vi "AutoRepScan.vi"() -> ()   [LabVIEW 2022 SP3]
uses:
  Control_AutoRepScan.ctl
  <vilib>/Utility/sysdir.llb/System Directory Type.ctl
  Peripherals/ActionEngineEnum(V2).ctl
  Peripherals/Control_ZurichAE.ctl
  <vilib>/DAQmx/read.llb/DAQmx Read (Counter U32 1Chan 1Samp).vi
  <vilib>/DAQmx/create/channels.llb/DAQmx Create Channel (CI-Count Edges).vi
  <vilib>/DAQmx/miscellaneous.llb/DAQmx Fill In Error Info.vi
  <resource>/objmgr/daqmx.rc
  C:/Users/mnopl/Desktop/Software/mnOPSuite/PRISM/Thorlabs.MotionControl.Controls.dll
  Thorlabs.MotionControl.Controls.dll
panel:
  in  "HeNe Vosc":cluster{"Node 1 (V)":dbl, "Node 2 (V)":dbl}={"Node 1 (V)"=0.04852, "Node 2 (V)"=0.07}
  in  "Do replicate on \"configure\"?":bool=TRUE
  out "Duration of scans":dbl(graph)=55.78836666666667
  in  "Timeout (min.)":dbl=1000.0
  out "PSHet V Oscillation vs. Wavelength":cluster{dbl[], dbl[]}(graph)={[3.16, 2.5200000000000005, 2.8400000000000003], [0.10222000000000002, 0.08074, 0.08074]}
  out "Current wavelength (microns)":dbl=2.8400000000000003
  in  "Replication wait time (s)":i32=2
  out "dWavelength/drep":dbl=0.32000000000000006
  in  "Default Zurich XY gain":dbl=100.0
  in  "Compromise Vosc to HeNeStab":bool=TRUE
  in  "Starting wavelength (microns)":dbl=2.2
  in  "Configure scan":bool
  out "Kinesis Errors":errorcluster
  out "dKinesis/dRep":dbl=0.010000000000000142
  in  "Ending Kinesis Pos.":dbl=12.38
  in  "Starting Kinesis Pos.":dbl=12.33
  in  "KCubeStepperControl":refnum<k24>(container)
  out "Scans Completed":bool
  in  "Manually increment counter":bool
  out "DAQ errors":errorcluster
  out "Digital counter":i32
  in  "Trigger Edge":i32(ring)=10171 items=["Rising"=10280, "Falling"=10171]
  in  "Scan (frame) trigger":tag="/Dev1/PFI1"
  in  "TTL control\nactive":bool
  out "Scans active":bool
  out "Python errors":errorcluster
  out "Zurich errors":errorcluster
  out "Current PSHet Osc":dbl=0.08074
  out "Number of scans":i32=3
  out "dOsc/drep":dbl=0.009600000000000001
  in  "Ending PSHet Osc":dbl=0.114
  in  "Starting PSHet Osc":dbl=0.066
  in  "Zurich Address":string="DEV1925"
  out "Latest alpha command":string="@rep load 2"
  out "# Scans completed":i32=3
  out "Current status":string="Awaiting command..."
  in  "Halt program":bool
  in  "Cancel Button":bool
  out "Time elapsed this scan (min)":dbl
  out "Time for last scan (min)":dbl
  in  "Current replication":i32=3
  in  "Execute Sequence":bool
  in  "Replicate to #":i32=5 min=0 max=49
  in  "Replicate from #":i32 min=0 max=49
  # "NOTE:  Replication list is assumed to increment uniformly in infrared *wavelength*, not uniformly in *frequency*."
  # "These should be a nearest pair of Vosc values at which HeNe-stab signal vanishes.\n(Updated 2025.05.08)"
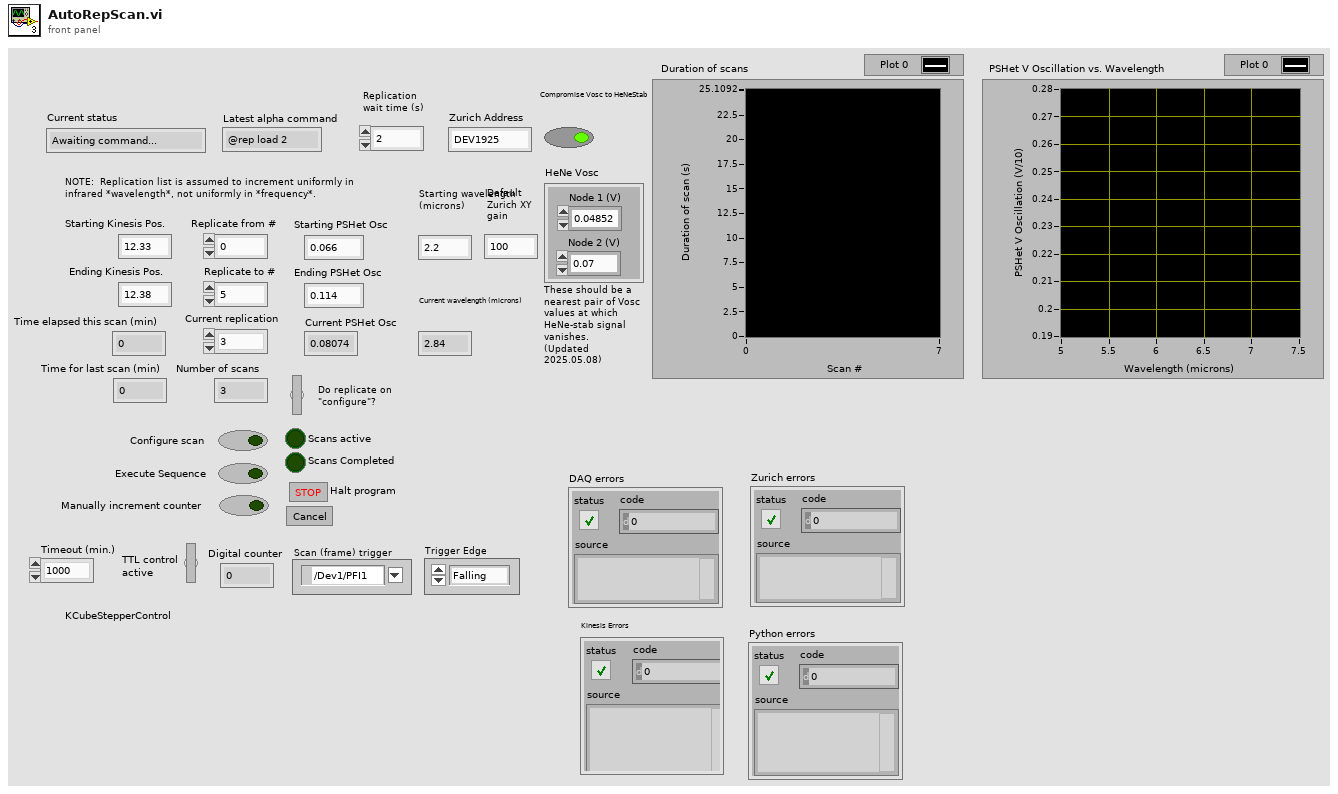
[diagram p1: front panel]
types:
  T1 = typedef "Control_ZurichAE.ctl" = enum16{"Initialize", "Set V oscillation", "Set XY gains", "Close", "Done"}
  T2 = typedef "ActionEngineEnum(V2).ctl" = enum16{"Open Connection", "IsSettingsInitialized? ", "Done", "Get Position", "Settings", "Home", "Move Absolute", "Move Relative", "Step", "Stop Action", "Close Connection"}
  T3 = typedef "System Directory Type.ctl" = i32
  T4 = typedef "Control_AutoRepScan.ctl" = enum16{"Sit Idle", "Configure scan", "Wait for scan", "Initialize", "Finalize", "Start DAQ control", "Poll DAQ control", "Stop DAQ control"}
  T5 = enum8{"Enabled", "Disabled", "Disabled and Grayed Out"}
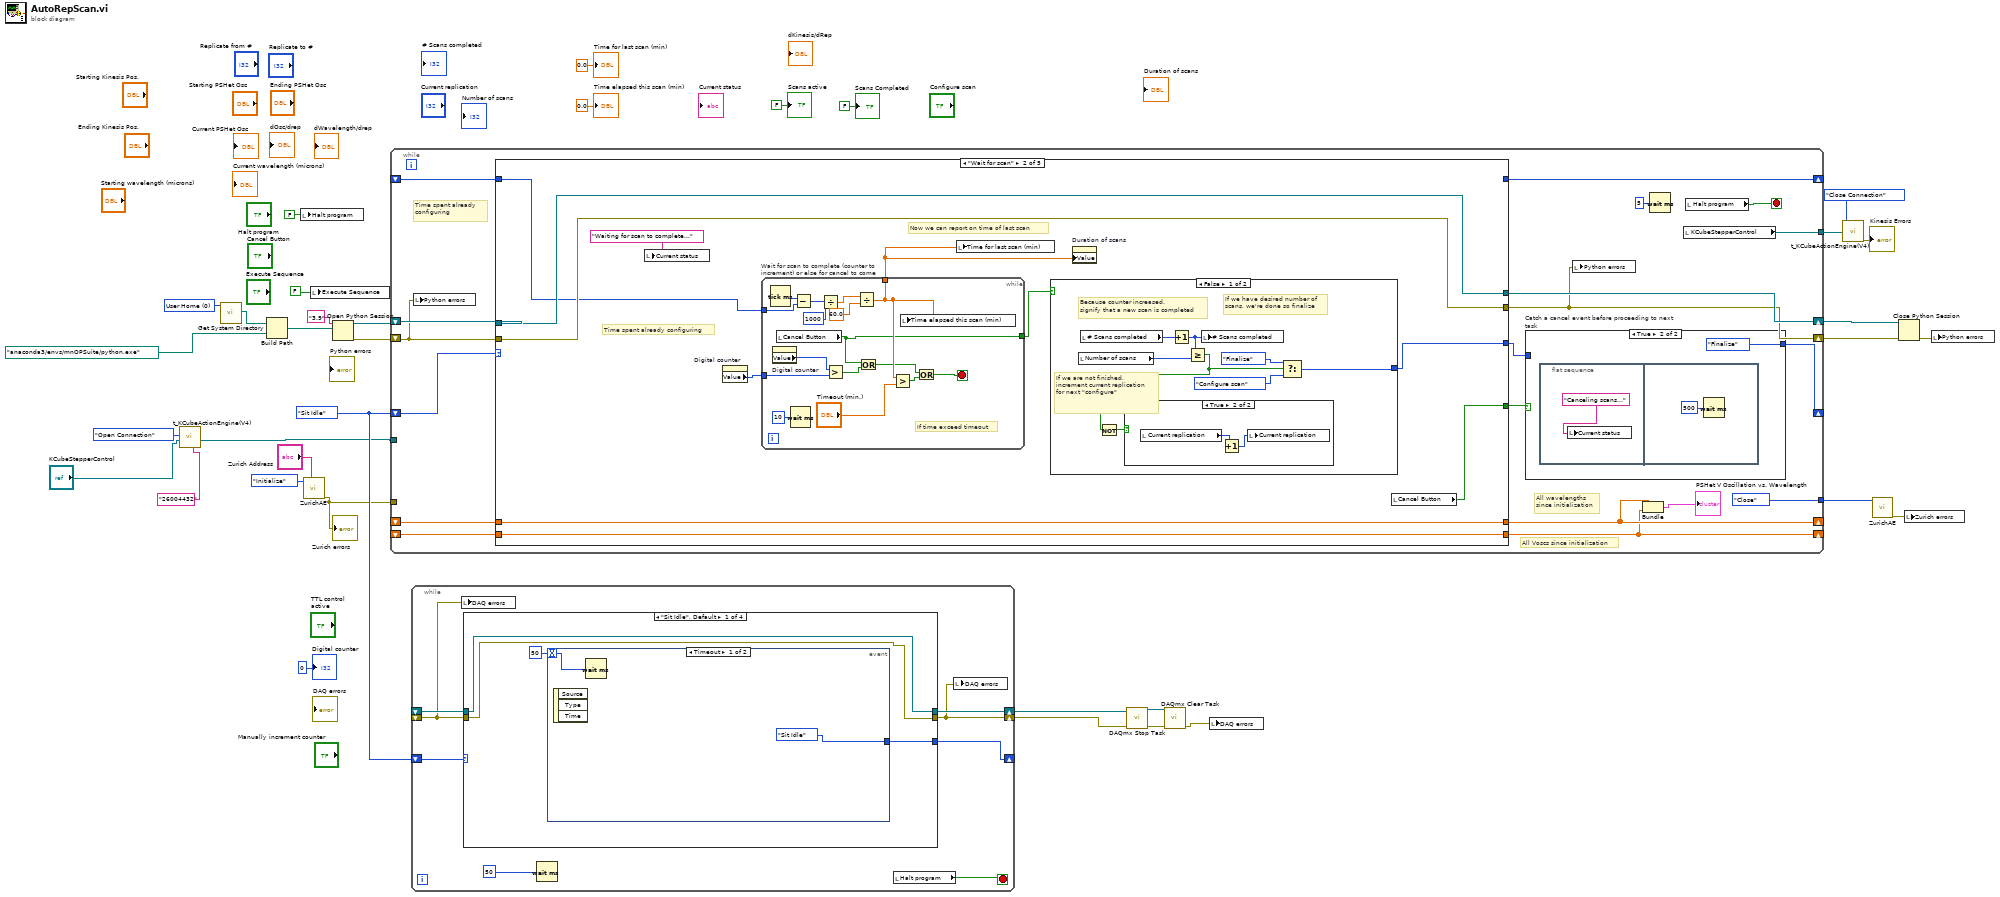
[diagram p0: block diagram]
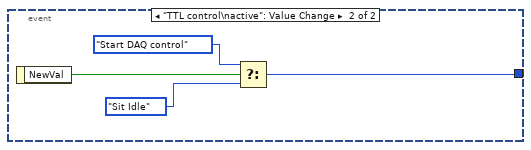
[diagram p2: hidden frame]
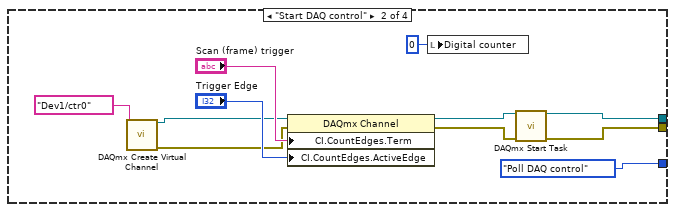
[diagram p3: hidden frame]
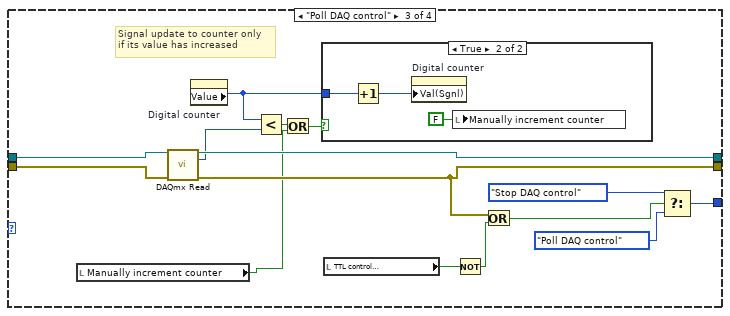
[diagram p4: hidden frame]
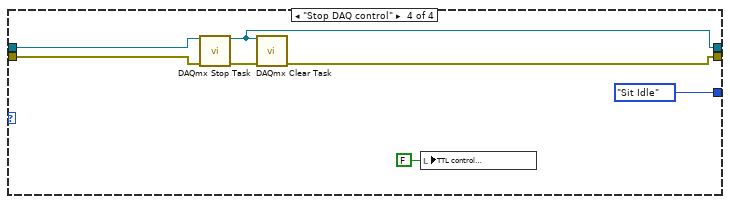
[diagram p6: hidden frame]
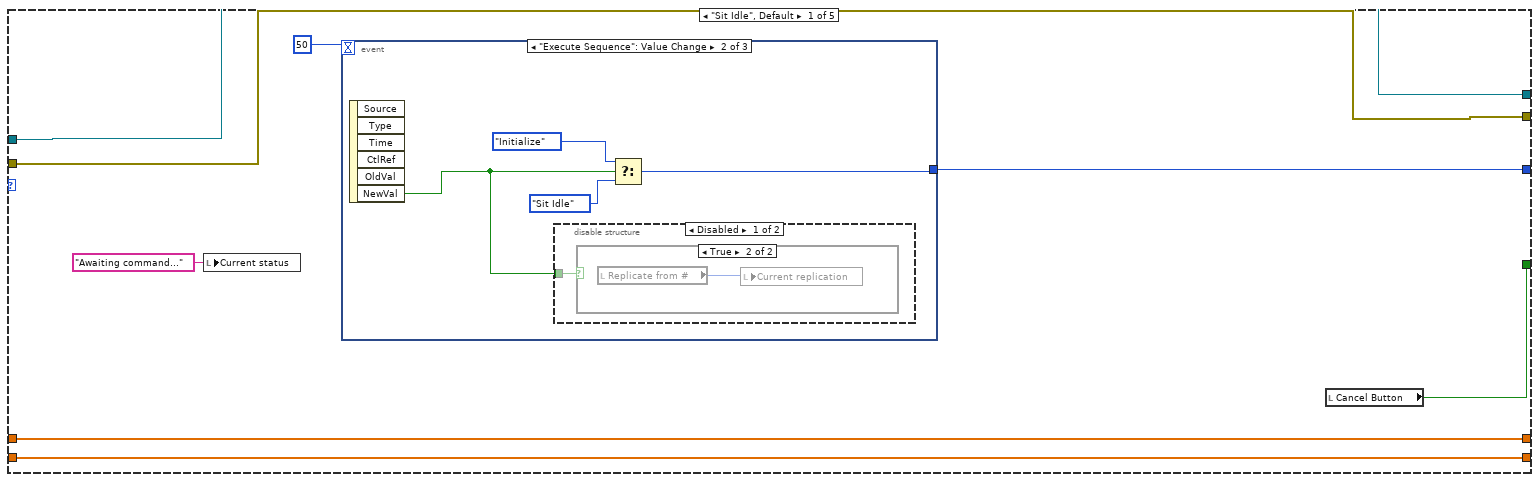
[diagram p8: hidden frame]
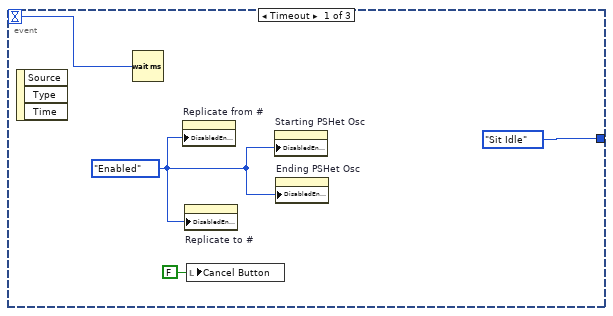
[diagram p9: hidden frame]
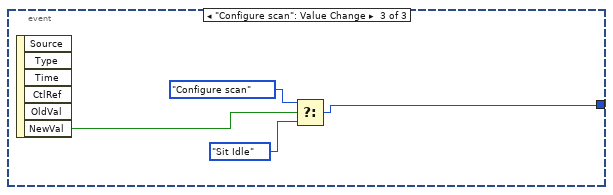
[diagram p12: hidden frame]
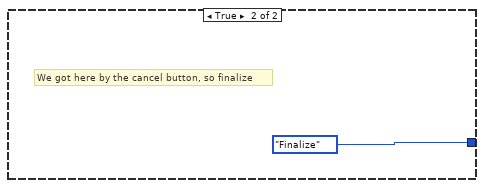
[diagram p14: hidden frame]
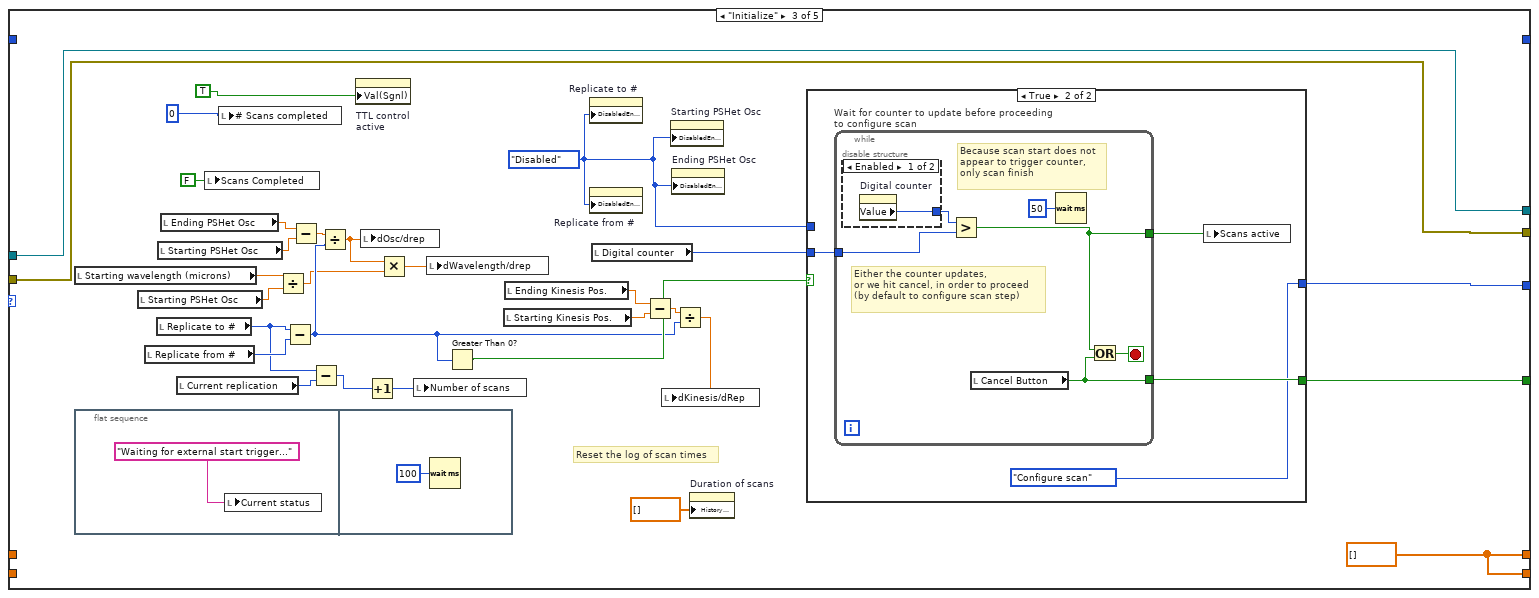
[diagram p15: hidden frame]
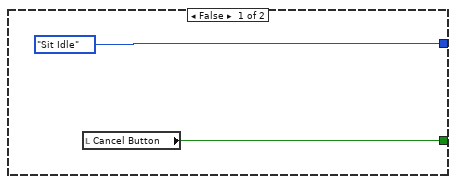
[diagram p16: hidden frame]
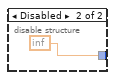
[diagram p17: hidden frame]
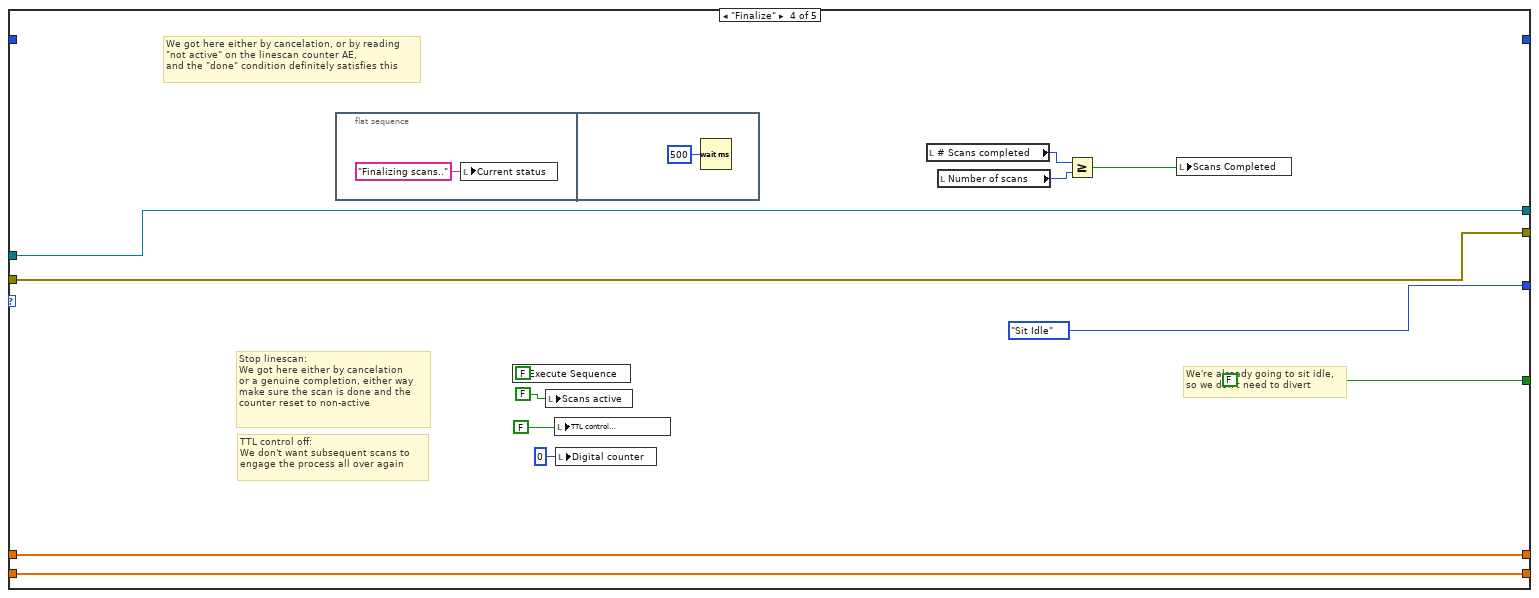
[diagram p18: hidden frame]
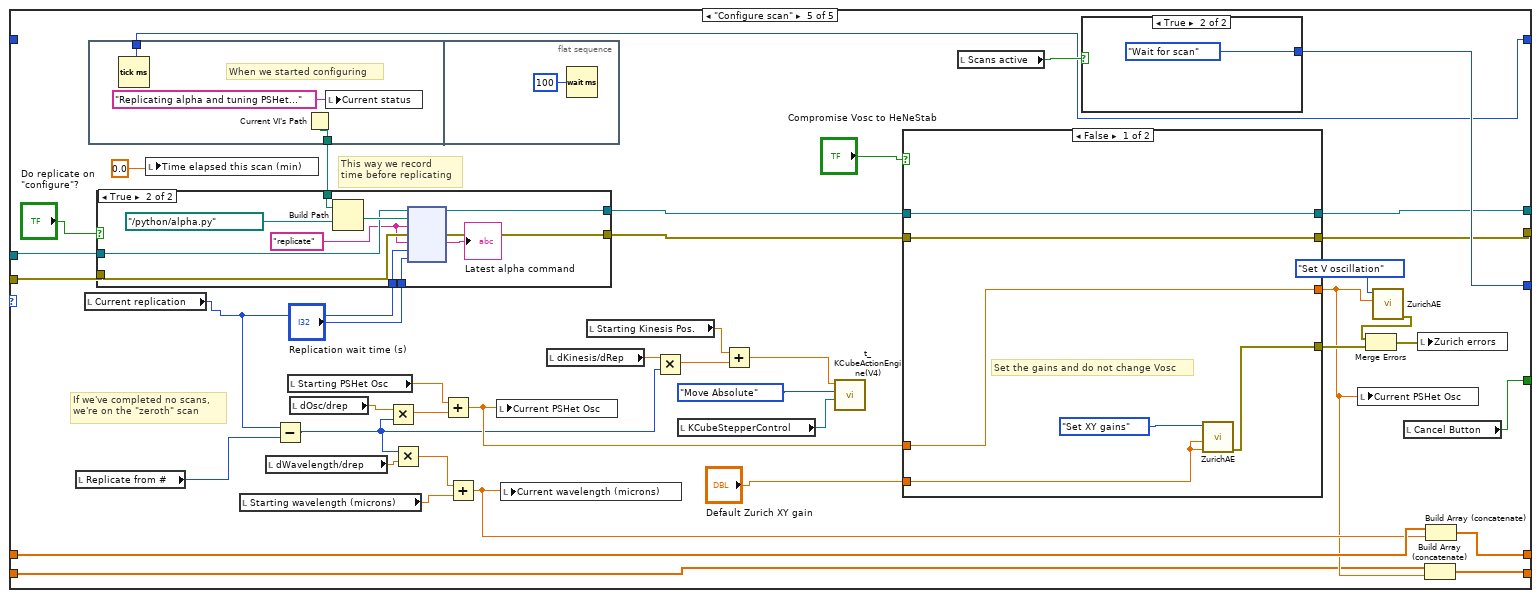
[diagram p19: hidden frame]
diagram:
  w34 = T3 0 items=["User Home"=0, "User Desktop"=1, "User Documents"=2, "User Application Data"=3, "User Preferences"=4, "User Temporary"=5, "Public Documents"=6, "Public Application Data"=7, "Public Preferences"=8, "Public Cache"=13, "System Core Libraries"=9, "System Installed Libraries"=10, "Application Files"=11, "Boot Volume Root"=12] ("system directory type")
  w23 = Control_AutoRepScan."Sit Idle"
  n1 = call "t_KCubeActionEngine(V4).vi"("SerialNumber"="26004432", "KCubeStepperControl"="KCubeStepperControl", "Action"=ActionEngineEnum(V2)."Open Connection") -> ("KCubeStepperControl Out"=w9:refnum<k24>)  [unwired: 5 in, 3 out]
  n2 = call <vilib>:"Get System Directory.vi"("system directory type"=w34) -> ("system directory"=w33:path)  [unwired: 10 in]
  n3 = Build Path(base path=w33, name or relative path=path "anaconda3/envs/mnOPSuite/python.exe") -> (appended path=w31:path)
  n4 = local write "Halt program"(FALSE ("Halt program")) -> ()
  n5 = call "ZurichAE.vi"("zi Address"="Zurich Address", "Action"=Control_ZurichAE."Initialize") -> ("Zurich Errors"=w3:errorcluster)  [unwired: 9 in]
  "Zurich errors" <- w3
  n6 = local write "Execute Sequence"(FALSE ("Execute")) -> ()
  n7 = Open Python Session(python version="3.9", python path=w31) -> (session out=w27:refnum<k35>, error out=w28:errorcluster)  [unwired: 1 in]
  n8 = while {
    shift-right: [w51] -> _
    shift-left: w23 -> [w54]
    shift-right: [w50] -> w30
    shift-left: w27 -> [w49]
    shift-right: [w46] -> w29
    shift-left: w28 -> [w47]
    tunnel: w9 -> [_]
    tunnel: [w44] -> w8
    tunnel: w3 -> [_]
    tunnel: [Control_ZurichAE."Close" ("Action")] -> w2
    shift-right: [w39] -> _
    shift-left: _ -> [w42]
    shift-right: [w38] -> _
    shift-left: _ -> [w41]
    shift-right: [w37] -> _
    shift-left: _ -> [w36]
    stop <- w53 stop-if-true
    # "Time spent already configuring"
    # "All Voscs since initialization"
    # "All wavelengths\nsince initialization"
    n9 = local write "Python errors"(w47) -> ()
    n10 = case shown="\"Wait for scan\"" w54 {
      tunnel: [w66 w85 w148 Control_AutoRepScan."Sit Idle" w216] -> w52
      tunnel: w47 -> [w63 w89 w140 w176 w220]
      tunnel: w49 -> [w64 w90 w141 w177 w221]
      tunnel: [w64 w90 w141 w177 w198] -> w50
      tunnel: [w63 w89 w140 w176 w196] -> w46
      tunnel: [w62 w91 w142 FALSE w215] -> w48
      tunnel: [w60 w84 w124 w166 w189] -> w39
      tunnel: [w59 w83 w124 w165 w186] -> w38
      tunnel: w42 -> [w60 w84 _ w166 w191]
      tunnel: w41 -> [w59 w83 _ w165 w187]
      tunnel: [_ _ _ _ w185] -> w37
      tunnel: w36 -> [_ w81 _ _ _]
      frame "Sit Idle", Default {
        n11 = local write "Current status"("Awaiting command..." ("Current status")) -> ()
        n12 = event shown="[1] \"Execute Sequence\": Value Change" {
          selector: _ -> [_ _ _]
          dyn-events: _ -> [_ _ _]
          timeout: 50 -> [w67 _ _]
          tunnel: [Control_AutoRepScan."Sit Idle" w73 w77] -> w66
          event Timeout {
            w69 = T5."Enabled" ("Disabled")
            n13 = event-data() -> ()  [unwired: 1 in, 3 out]
            n14 = Wait (ms)(milliseconds to wait=w67) -> ()  [unwired: 1 out]
            n15 = property on="Replicate from #" class="DigNum (strict)"("DisabledEnum"=w69) -> ()  [unwired: 2 in, 2 out]
            n16 = property on="Replicate to #" class="DigNum (strict)"("DisabledEnum"=w69) -> ()  [unwired: 2 in, 2 out]
            n17 = local write "Cancel Button"(FALSE ("Cancel Button")) -> ()
            n18 = property on="Starting PSHet Osc" class="DigNum (strict)"("DisabledEnum"=w69) -> ()  [unwired: 2 in, 2 out]
            n19 = property on="Ending PSHet Osc" class="DigNum (strict)"("DisabledEnum"=w69) -> ()  [unwired: 2 in, 2 out]
          }
          event "Execute Sequence": Value Change {
            n20 = event-data() -> ("NewVal"=w71:bool)  [unwired: 1 in, 5 out]
            n21 = disable-structure shown="Disabled" {
              disable-tunnel: w71 -> [w75 _]
              frame Disabled {
                n22 = case shown="True" w75 {
                  frame False {
                  }
                  frame True {
                    n23 = local read "Replicate from #"() -> (w76:i32)
                    n24 = local write "Current replication"(w76) -> ()
                  }
                }
              }
              frame Enabled {
              }
            }
            n25 = Select(t=Control_AutoRepScan."Initialize", s=w71, f=Control_AutoRepScan."Sit Idle") -> (s? t:f=w73:T4)
          }
          event "Configure scan": Value Change {
            n26 = event-data() -> ("NewVal"=w80:bool)  [unwired: 1 in, 5 out]
            n27 = Select(t=Control_AutoRepScan."Configure scan", s=w80, f=Control_AutoRepScan."Sit Idle") -> (s? t:f=w77:T4)
          }
        }
        n28 = local read "Cancel Button"() -> (w62:bool)
      }
      frame "Wait for scan" {
        # "Time spent already configuring"
        # "Now we can report on time of last scan"
        n29 = local write "Current status"("Waiting for scan to complete..." ("Current status")) -> ()
        n30 = property on="Digital counter" class="DigNum (strict)"() -> ("Value"=w87:i32)  [unwired: 2 in, 2 out]
        n31 = while "Wait for scan to complete (counter to increment) or else for cancel to come" {
          tunnel: w81 -> [w112]
          tunnel: [w108] -> w82
          tunnel: w87 -> [w115]
          tunnel: [w104] -> w86
          stop <- w106 stop-if-true
          # "If time exceed timeout"
          n32 = Tick Count (ms)() -> (millisecond timer value=w113:u32)
          n33 = property on="Digital counter" class="DigNum (strict)"() -> ("Value"=w116:i32)  [unwired: 2 in, 2 out]
          n34 = local read "Cancel Button"() -> (w104:bool)
          n35 = Wait (ms)(milliseconds to wait=u32 10) -> ()  [unwired: 1 out]
          n36 = Subtract(x=w113, y=w112) -> (x-y=w114:u32)
          n37 = Divide(x=w114, y=u32 1000) -> (x/y=w111:dbl)
          n38 = Greater?(x=w116, y=w115) -> (0:w105:bool)
          n39 = Divide(x=w111, y=60.0) -> (x/y=w108:dbl)
          n40 = Or(x=w104, y=w105) -> (x .or. y?=w107:bool)
          n41 = Greater?(x=w108, y="Timeout (min.)") -> (0:w109:bool)
          n42 = local write "Time elapsed this scan (min)"(w108) -> ()
          n43 = Or(x=w107, y=w109) -> (x .or. y?=w106:bool)
        }
        n44 = local write "Time for last scan (min)"(w82) -> ()
        n45 = case shown="False" w86 {
          tunnel: [w94 Control_AutoRepScan."Finalize"] -> w85
          frame False {
            # "If we are not finished, increment current replication for next \"configure\""
            # "If we have desired number of\nscans, we're done so finalize"
            # "Because counter increased,\nsignify that a new scan is completed"
            n46 = local read "Number of scans"() -> (w98:i32)
            n47 = local read "# Scans completed"() -> (w99:i32)
            n48 = Increment(x=w99) -> (x+1=w97:i32)
            n49 = Greater Or Equal?(x=w97, y=w98) -> (x >= y?=w93:bool)
            n50 = Not(x=w93) -> (.not. x?=w92:bool)
            n51 = case shown="True" w92 {
              frame False {
              }
              frame True {
                n52 = local read "Current replication"() -> (w100:i32)
                n53 = Increment(x=w100) -> (x+1=w101:i32)
                n54 = local write "Current replication"(w101) -> ()
              }
            }
            n55 = local write "# Scans completed"(w97) -> ()
            n56 = Select(t=Control_AutoRepScan."Finalize", s=w93, f=Control_AutoRepScan."Configure scan") -> (s? t:f=w94:T4)
          }
          frame True {
            # "We got here by the cancel button, so finalize"
          }
        }
        n57 = property on="Duration of scans" class="WFChart (strict)"("Value"=w82) -> ()  [unwired: 2 in, 2 out]
        n58 = local read "Cancel Button"() -> (w91:bool)
      }
      frame "Initialize" {
        w124 = dbl[] []
        w144 = T5."Disabled" ("Disabled")
        # "Reset the log of scan times"
        n59 = local read "Starting wavelength (microns)"() -> (w123:dbl)
        n60 = flat-sequence {
          frame #0 {
            n61 = local write "Current status"("Waiting for external start trigger..." ("Current status")) -> ()
          }
          frame #1 {
            n62 = Wait (ms)(milliseconds to wait=u32 100) -> ()  [unwired: 1 out]
          }
        }
        n63 = local read "Starting PSHet Osc"() -> (w129:dbl)
        n64 = local read "Replicate from #"() -> (w126:i32)
        n65 = local read "Replicate to #"() -> (w121:i32)
        n66 = local read "Starting PSHet Osc"() -> (w145:dbl)
        n67 = local read "Ending PSHet Osc"() -> (w146:dbl)
        n68 = local read "Current replication"() -> (w120:i32)
        n69 = local write "Scans Completed"(FALSE ("Scans Completed")) -> ()
        n70 = local write "# Scans completed"(0 ("# Scans completed")) -> ()
        n71 = Divide(x=w123, y=w129) -> (x/y=w128:dbl)
        n72 = Subtract(x=w121, y=w126) -> (x-y=w134:i32)
        n73 = Subtract(x=w146, y=w145) -> (x-y=w143:dbl)
        n74 = Subtract(x=w121, y=w120) -> (x-y=w119:i32)
        n75 = Divide(x=w143, y=w134) -> (x/y=w127:dbl)
        n76 = property on="TTL control\nactive" class="Bool (strict)"("Val(Sgnl)"=TRUE ("TTL control\nactive")) -> ()  [unwired: 2 in, 2 out]
        n77 = local write "dOsc/drep"(w127) -> ()
        n78 = Increment(x=w119) -> (x+1=w139:i32)
        n79 = Multiply(x=w127, y=w128) -> (x*y=w125:dbl)
        n80 = local write "Number of scans"(w139) -> ()
        n81 = local write "dWavelength/drep"(w125) -> ()
        n82 = Greater Than 0?(x=w134) -> (x > 0?=w147:bool)
        n83 = local read "Starting Kinesis Pos."() -> (w130:dbl)
        n84 = local read "Ending Kinesis Pos."() -> (w131:dbl)
        n85 = property on="Replicate to #" class="DigNum (strict)"("DisabledEnum"=w144) -> ()  [unwired: 2 in, 2 out]
        n86 = property on="Replicate from #" class="DigNum (strict)"("DisabledEnum"=w144) -> ()  [unwired: 2 in, 2 out]
        n87 = local read "Digital counter"() -> (w138:i32)
        n88 = Subtract(x=w131, y=w130) -> (x-y=w133:dbl)
        n89 = property on="Starting PSHet Osc" class="DigNum (strict)"("DisabledEnum"=w144) -> ()  [unwired: 2 in, 2 out]
        n90 = property on="Ending PSHet Osc" class="DigNum (strict)"("DisabledEnum"=w144) -> ()  [unwired: 2 in, 2 out]
        n91 = Divide(x=w133, y=w134) -> (x/y=w132:dbl)
        n92 = local write "dKinesis/dRep"(w132) -> ()
        n93 = property on="Duration of scans" class="WFChart (strict)"("History Data"=dbl[] []) -> ()  [unwired: 2 in, 2 out]
        n94 = case shown="True" w147 {
          tunnel: [Control_AutoRepScan."Sit Idle" Control_AutoRepScan."Configure scan"] -> w148
          tunnel: w144 -> [_ _]
          tunnel: [w151 w155] -> w142
          tunnel: w138 -> [_ w156]
          frame False {
            n95 = local read "Cancel Button"() -> (w151:bool)
          }
          frame True {
            n96 = while "Wait for counter to update before proceeding to configure scan" {
              tunnel: w156 -> [w161]
              tunnel: [w159] -> w155
              tunnel: [w157] -> w153
              stop <- w158 stop-if-true
              # "Because scan start does not\nappear to trigger counter, \nonly scan finish"
              # "Either the counter updates,\nor we hit cancel, in order to proceed\n(by default to configure scan step)"
              n97 = disable-structure shown="Enabled" {
                disable-tunnel: [w163 inf] -> w162
                frame Enabled {
                  n98 = property on="Digital counter" class="DigNum (strict)"() -> ("Value"=w163:i32)  [unwired: 2 in, 2 out]
                }
                frame Disabled {
                }
              }
              n99 = Greater?(x=w162, y=w161) -> (0:w157:bool)
              n100 = local read "Cancel Button"() -> (w159:bool)
              n101 = Wait (ms)(milliseconds to wait=u32 50) -> ()  [unwired: 1 out]
              n102 = Or(x=w157, y=w159) -> (x .or. y?=w158:bool)
            }
            n103 = local write "Scans active"(w153) -> ()
          }
        }
      }
      frame "Finalize" {
        # "We're already going to sit idle,\nso we don't need to divert"
        # "We got here either by cancelation, or by reading\n\"not active\" on the linescan counter AE,\nand the \"done\" condition definitely satisfies this"
        # "TTL control off:\nWe don't want subsequent scans to\nengage the process all over again"
        # "Stop linescan:\nWe got here either by cancelation\nor a genuine completion, either way\nmake sure the scan is done and the\ncounter reset to non-active"
        n104 = flat-sequence {
          frame #0 {
            n105 = local write "Current status"("Finalizing scans.." ("Current status")) -> ()
          }
          frame #1 {
            n106 = Wait (ms)(milliseconds to wait=u32 500) -> ()  [unwired: 1 out]
          }
        }
        n107 = local write "Execute Sequence"(FALSE ("Execute")) -> ()
        n108 = local write "Scans active"(FALSE ("Stop linescan")) -> ()
        n109 = local write "TTL control\nactive"(FALSE ("TTL Control Active")) -> ()
        n110 = local write "Digital counter"(0 ("Digital counter")) -> ()
        n111 = local read "# Scans completed"() -> (w169:i32)
        n112 = local read "Number of scans"() -> (w168:i32)
        n113 = Greater Or Equal?(x=w169, y=w168) -> (x >= y?=w167:bool)
        n114 = local write "Scans Completed"(w167) -> ()
      }
      frame "Configure scan" {
        # "This way we record\ntime before replicating"
        # "If we've completed no scans,\nwe're on the \"zeroth\" scan"
        n115 = local read "Replicate from #"() -> (w180:i32)
        n116 = local read "Current replication"() -> (w182:i32)
        n117 = flat-sequence {
          tunnel: [w268] -> w185
          tunnel: [w267] -> w184
          frame #0 {
            # "When we started configuring"
            n118 = Tick Count (ms)() -> (millisecond timer value=w268:u32)
            n119 = Current VI's Path() -> (path=w267:path)
            n120 = local write "Current status"("Replicating alpha and tuning PSHet..." ("Current status")) -> ()
          }
          frame #1 {
            n121 = Wait (ms)(milliseconds to wait=u32 100) -> ()  [unwired: 1 out]
          }
        }
        n122 = case shown="True" "Do replicate on \"configure\"?" {
          tunnel: w221 -> [w222 w232]
          tunnel: w220 -> [w223 w231]
          tunnel: "Replication wait time (s)" -> [_ w228]
          tunnel: [w222 w227] -> w199
          tunnel: [w223 w226] -> w197
          tunnel: w184 -> [_ w225]
          tunnel: w182 -> [_ w224]
          frame False {
          }
          frame True {
            w230 = "replicate" ("function name")
            n123 = Build Path(base path=w225, name or relative path=path "../python/alpha.py") -> (appended path=w233:path)
            n124 = node(w232, w233, w230, w231, w230, w224, w228) -> (w227:refnum<k35>, w226:errorcluster, →"Latest alpha command":string)  [unwired: 2 in, 2 out]
          }
        }
        n125 = local write "Time elapsed this scan (min)"(0.0 ("Time elapsed this scan (s)")) -> ()
        n126 = local read "Starting wavelength (microns)"() -> (w205:dbl)
        n127 = local read "dWavelength/drep"() -> (w203:dbl)
        n128 = Subtract(x=w182, y=w180) -> (x-y=w181:i32)
        n129 = local read "Starting PSHet Osc"() -> (w218:dbl)
        n130 = local read "dOsc/drep"() -> (w219:dbl)
        n131 = Multiply(x=w219, y=w181) -> (x*y=w217:dbl)
        n132 = Multiply(x=w181, y=w203) -> (x*y=w204:dbl)
        n133 = Add(x=w218, y=w217) -> (x+y=w201:dbl)
        n134 = Add(x=w204, y=w205) -> (x+y=w190:dbl)
        n135 = local write "Current PSHet Osc"(w201) -> ()
        n136 = local write "Current wavelength (microns)"(w190) -> ()
        n137 = local read "dKinesis/dRep"() -> (w210:dbl)
        n138 = local read "Starting Kinesis Pos."() -> (w209:dbl)
        n139 = Multiply(x=w210, y=w181) -> (x*y=w211:dbl)
        n140 = local read "KCubeStepperControl"() -> (w212:refnum<k24>)
        n141 = Add(x=w209, y=w211) -> (x+y=w208:dbl)
        n142 = call "t_KCubeActionEngine(V4).vi"("KCubeStepperControl"=w212, "Action"=ActionEngineEnum(V2)."Move Absolute", "Input Position"=w208) -> ()  [unwired: 5 in, 4 out]
        n143 = case shown="False" "Compromise Vosc to HeNeStab" {
          tunnel: w201 -> [w240 w257]
          tunnel: "Default Zurich XY gain" -> [w238 w244]
          tunnel: w199 -> [w236 w262]
          tunnel: [w236 w261] -> w198
          tunnel: w197 -> [w235 w260]
          tunnel: [w235 w259] -> w196
          tunnel: [w240 w254] -> w188
          tunnel: [w237 w248] -> w193
          frame False {
            # "Set the gains and do not change Vosc"
            n144 = call "ZurichAE.vi"("Y gain"=w238, "X gain"=w238, "Action"=Control_ZurichAE."Set XY gains") -> ("Zurich Errors"=w237:errorcluster)  [unwired: 8 in]
          }
          frame True {
            # "V_ideal"
            # "Recompute a compromise \nset of parameters between\ntuned laser and HeNe stab"
            # "Vcompromise"
            n145 = Unbundle By Name("HeNe Vosc") -> ("Node 1 (V)"=w242:dbl, "Node 2 (V)"=w241:dbl)
            n146 = Current VI's Path() -> (path=w247:path)
            n147 = Build Path(base path=w247, name or relative path=path "../python/zurich.py") -> (appended path=w245:path)
            n148 = node(w262, w245, "get_compromise_V_and_XYgains" ("function name"), w260, dbl[] [0.0], w257, w242, w241, w244) -> (w261:refnum<k35>, w259:errorcluster, w252:dbl[])  [unwired: 4 in, 2 out]
            n149 = Index Array(array=w252, index=1) -> (element=w250:dbl)
            n150 = Index Array(array=w252, index=2) -> (element=w249:dbl)
            n151 = call "ZurichAE.vi"("Y gain"=w249, "X gain"=w250, "Action"=Control_ZurichAE."Set XY gains") -> ("Zurich Errors"=w248:errorcluster)  [unwired: 8 in]
            n152 = Index Array(array=w252, index=0) -> (element=w254:dbl)
          }
        }
        n153 = local read "Scans active"() -> (w207:bool)
        n154 = case shown="True" w207 {
          tunnel: [Control_AutoRepScan."Sit Idle" Control_AutoRepScan."Wait for scan"] -> w216
          frame False {
            n155 = local write "Configure scan"(FALSE ("Configure scan")) -> ()
          }
          frame True {
          }
        }
        n156 = local write "Current PSHet Osc"(w188) -> ()
        n157 = call "ZurichAE.vi"("V oscillation"=w188, "Action"=Control_ZurichAE."Set V oscillation") -> ("Zurich Errors"=w194:errorcluster)  [unwired: 9 in]
        n158 = Merge Errors(w194, w193) -> (w192:errorcluster)
        n159 = local read "Cancel Button"() -> (w215:bool)
        n160 = local write "Zurich errors"(w192) -> ()
        n161 = Build Array (concatenate)(w187, w188) -> (w186:dbl[])
        n162 = Build Array (concatenate)(w191, w190) -> (w189:dbl[])
      }
    }
    n163 = case "Catch a cancel event before proceeding to next task" shown="True" w48 {
      tunnel: w52 -> [w55 _]
      tunnel: [w55 Control_AutoRepScan."Finalize"] -> w51
      frame False {
      }
      frame True {
        n164 = flat-sequence {
          frame #0 {
            n165 = local write "Current status"("Canceling scans..." ("Current status")) -> ()
          }
          frame #1 {
            n166 = Wait (ms)(milliseconds to wait=u32 500) -> ()  [unwired: 1 out]
          }
        }
      }
    }
    n167 = local write "Python errors"(w46) -> ()
    n168 = Bundle(w39, w38) -> (→"PSHet V Oscillation vs. Wavelength":cluster{dbl[], dbl[]})  [unwired: 1 in]
    n169 = Wait (ms)(milliseconds to wait=u32 5) -> ()  [unwired: 1 out]
    n170 = local read "KCubeStepperControl"() -> (w44:refnum<k24>)
    n171 = local read "Halt program"() -> (w53:bool)
  }
  n172 = while {
    shift-right: [w275] -> _
    shift-left: w23 -> [w276]
    shift-right: [w272] -> w19
    shift-left: _ -> [w271]
    shift-right: [w274] -> w20
    shift-left: _ -> [w273]
    stop <- w278 stop-if-true
    n173 = local write "DAQ errors"(w271) -> ()
    n174 = case shown="\"Sit Idle\", Default" w276 {
      tunnel: [w282 Control_AutoRepScan."Poll DAQ control" w304 Control_AutoRepScan."Sit Idle"] -> w275
      tunnel: [w280 w290 w311 w321] -> w274
      tunnel: [w279 w289 w308 w320] -> w272
      tunnel: w273 -> [w280 _ w313 w323]
      tunnel: w271 -> [w279 _ w312 w322]
      frame "Sit Idle", Default {
        n175 = event shown="[0] Timeout" {
          selector: _ -> [_ _]
          dyn-events: _ -> [_ _]
          timeout: 50 -> [w283 _]
          tunnel: [Control_AutoRepScan."Sit Idle" w285] -> w282
          event Timeout {
            n176 = event-data() -> ()  [unwired: 1 in, 3 out]
            n177 = Wait (ms)(milliseconds to wait=w283) -> ()  [unwired: 1 out]
          }
          event "TTL control\nactive": Value Change {
            n178 = event-data() -> ("NewVal"=w288:bool)  [unwired: 1 in]
            n179 = Select(t=Control_AutoRepScan."Start DAQ control", s=w288, f=Control_AutoRepScan."Sit Idle") -> (s? t:f=w285:T4)
          }
        }
      }
      frame "Start DAQ control" {
        n180 = call-poly <vilib>:"DAQmx Create Virtual Channel.vi"("counter"=tag "Dev1/ctr0") -> ("task out"=w296:refnum<k21>, "error out"=w295:errorcluster)  [unwired: 13 in]
        n181 = property class="DAQmx Channel"(reference=w296, error in=w295, "CI.CountEdges.Term"="Scan (frame) trigger", "CI.CountEdges.ActiveEdge"="Trigger Edge") -> (reference out=w292:refnum<k21>, error out=w291:errorcluster)
        n182 = local write "Digital counter"(0 ("Digital counter")) -> ()
        n183 = call <vilib>:"DAQmx Start Task.vi"("task/channels in"=w292, "error in"=w291) -> ("task out"=w290:refnum<k21>, "error out"=w289:errorcluster)  [unwired: 12 in]
      }
      frame "Poll DAQ control" {
        # "Signal update to counter only\nif its value has increased"
        n184 = local read "Manually increment counter"() -> (w300:bool)
        n185 = call-poly <vilib>:"DAQmx Read.vi"("task/channels in"=w313, "error in"=w312) -> ("task out"=w311:refnum<k21>, "data"=w303:u32, "error out"=w308:errorcluster)  [unwired: 11 in]
        n186 = property on="Digital counter" class="DigNum (strict)"() -> ("Value"=w314:i32)  [unwired: 2 in, 2 out]
        n187 = Less?(x=w314, y=w303) -> (x < y?=w302:bool)
        n188 = Or(x=w302, y=w300) -> (x .or. y?=w301:bool)
        n189 = case shown="True" w301 {
          tunnel: w314 -> [_ w316]
          frame False {
          }
          frame True {
            n190 = Increment(x=w316) -> (x+1=w317:i32)
            n191 = property on="Digital counter" class="DigNum (strict)"("Val(Sgnl)"=w317) -> ()  [unwired: 2 in, 2 out]
            n192 = local write "Manually increment counter"(FALSE ("Manually increment counter")) -> ()
          }
        }
        n193 = local read "TTL control\nactive"() -> (w309:bool)
        n194 = Not(x=w309) -> (.not. x?=w307:bool)
        n195 = Or(x=w308, y=w307) -> (x .or. y?=w306:bool)
        n196 = Select(t=Control_AutoRepScan."Stop DAQ control", s=w306, f=Control_AutoRepScan."Poll DAQ control") -> (s? t:f=w304:T4)
      }
      frame "Stop DAQ control" {
        n197 = call <vilib>:"DAQmx Stop Task.vi"("task/channels in"=w323, "error in"=w322) -> ("task out"=w321:refnum<k21>, "error out"=w324:errorcluster)  [unwired: 12 in]
        n198 = call <vilib>:"DAQmx Clear Task.vi"("task in"=w321, "error in"=w324) -> ("error out"=w320:errorcluster)  [unwired: 13 in]
        n199 = local write "TTL control\nactive"(FALSE ("TTL control\nactive")) -> ()
      }
    }
    n200 = Wait (ms)(milliseconds to wait=50) -> ()  [unwired: 1 out]
    n201 = local read "Halt program"() -> (w278:bool)
    n202 = local write "DAQ errors"(w272) -> ()
  }
  n203 = call <vilib>:"DAQmx Stop Task.vi"("task/channels in"=w20, "error in"=w19) -> ("task out"=w21:refnum<k21>, "error out"=w22:errorcluster)  [unwired: 12 in]
  n204 = call <vilib>:"DAQmx Clear Task.vi"("task in"=w21, "error in"=w22) -> ("error out"=w15:errorcluster)  [unwired: 13 in]
  n205 = local write "DAQ errors"(w15) -> ()
  n206 = call "t_KCubeActionEngine(V4).vi"("KCubeStepperControl"=w8, "Action"=ActionEngineEnum(V2)."Close Connection") -> ("error out"=→"Kinesis Errors":errorcluster)  [unwired: 6 in, 3 out]
  n207 = call "ZurichAE.vi"("Action"=w2) -> ("Zurich Errors"=w1:errorcluster)  [unwired: 10 in]
  n208 = Close Python Session(session in=w30, error in=w29) -> (11:w24:errorcluster)
  n209 = local write "Zurich errors"(w1) -> ()
  n210 = local write "Python errors"(w24) -> ()
  "Time for last scan (min)" <- 0.0 ("Time for last scan (s)")
  "Time elapsed this scan (min)" <- 0.0 ("Time elapsed this scan (s)")
  "Scans active" <- FALSE ("Scan active")
  "Digital counter" <- 0 ("Digital counter")
  "Scans Completed" <- FALSE ("Scans Completed")
